vi "Render Template (Path).vi"(6 "Locals (None)":refnum<class "Value Tree.lvclass">, 8 "error in (no error)":errorcluster, 10 "Path":path, 11 "BasicTemplater in":refnum<class "BasicTemplater.lvclass">) -> (0 "error out":errorcluster, 2 "String":string, 3 "BasicTemplater out":refnum<class "BasicTemplater.lvclass">)   [LabVIEW 2020, in "HTTP Server.lvlib" / "BasicTemplater.lvclass"]
uses:
  BasicTemplater.lvclass
  Value Tree/Value Tree.lvclass
  BasicTemplater.lvclass/BasicTemplater.ctl
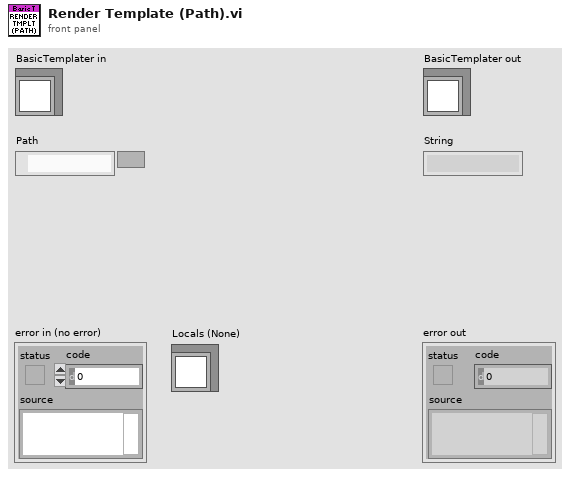
[diagram p1: front panel]
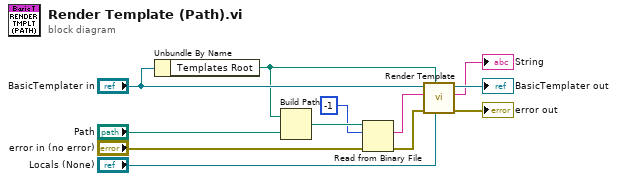
[diagram p0: block diagram]
diagram:
  n1 = Unbundle By Name("BasicTemplater in") -> ("Templates Root"=w6:path)
  n2 = Build Path(base path=w6, name or relative path="Path") -> (appended path=w11:path)
  n3 = Read from Binary File(8:"error in (no error)", 10:-1 ("count (1)"), 11:w11) -> (0:w3:errorcluster, 2:w5:string)  [unwired: 3 in, 2 out]
  n4 = call-dynamic "Render Template.vi"("Locals (None)"="Locals (None)", "Folder"=w6, "error in (no error)"=w3, "Template"=w5, "BasicTemplater in"="BasicTemplater in") -> ("error out"=→"error out":errorcluster, "Output"=→"String":string, "BasicTemplater out"=→"BasicTemplater out":refnum<class "BasicTemplater.lvclass">)  [unwired: 4 in]
